vi "mod_GetPolyphaseFilter.vi"(10 "# of zero crossings":i32=8, 11 "interpolation factor in":i32=512) -> (0 "effective filter length":i32=16, 1 "interpolation factor":i32=128, 2 "differencesBetweenCoeffs[]":dbl[](array[numeric]), 3 "scaledFilterCoefficients[]":dbl[](array[numeric]))   [LabVIEW 2020, in "niAMT.lvlib"]
uses:
  <vilib>/addons/Modulation/niAMT.lvlib
  nilvamt.dll
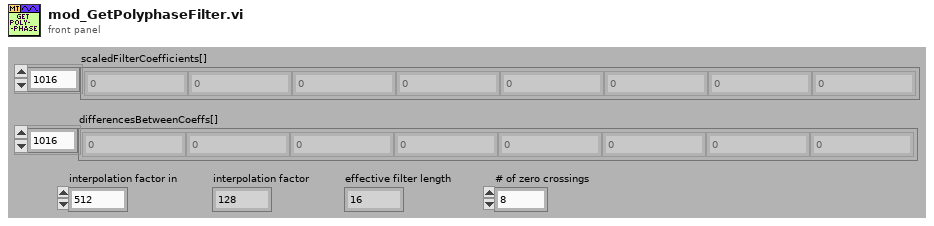
[diagram p1: front panel]
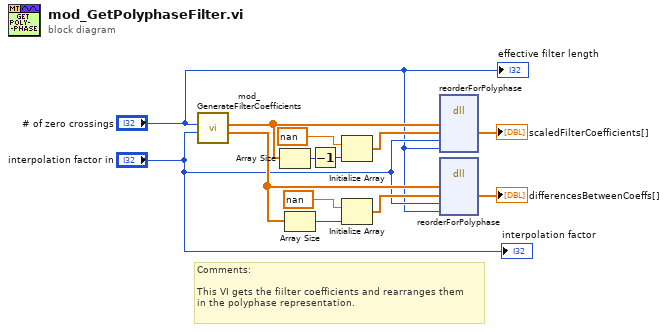
[diagram p0: block diagram]
diagram:
  # "Comments:\n\nThis VI gets the fiilter coefficients and rearranges them\nin the polyphase representation."
  n1 = call <vilib>:"mod_GenerateFilterCoefficients.vi"("interpolation factor"="interpolation factor in", "# of zero crossings"="# of zero crossings") -> ("Differences (scaled)"=w5:dbl[], "Filter Coefficients (scaled)"=w12:dbl[])  [unwired: 1 in, 7 out]
  n2 = Array Size(array=w12) -> (size(s)=w13:i32)
  n3 = Array Size(array=w5) -> (size(s)=w10:i32)
  n4 = Decrement(x=w13) -> (x-1=w1:i32)
  n5 = Initialize Array(nan ("element"), w1) -> (w11:dbl[])
  n6 = Initialize Array(nan ("element"), w10) -> (w4:dbl[])
  n7 = dll-call lib="nilvamt.*" fn="reorderForPolyphase"("arrayIn"=w12, "arrayOut"=w11, "interpolation factor"="interpolation factor in", "effective filter length"="# of zero crossings") -> ("arrayOut"=→"scaledFilterCoefficients[]":dbl[])  [unwired: 6 in, 3 out]
  n8 = dll-call lib="nilvamt.*" fn="reorderForPolyphase"("arrayIn"=w5, "arrayOut"=w4, "interpolation factor"="interpolation factor in", "effective filter length"="# of zero crossings") -> ("arrayOut"=→"differencesBetweenCoeffs[]":dbl[])  [unwired: 6 in, 3 out]
  "interpolation factor" <- "interpolation factor in"
  "effective filter length" <- "# of zero crossings"
